vi "Calib_Substring_code.vi"(0 "Inst type":T1=enum."Pressure Transducer") -> (1 "Substring Type":string, 2 "Read file":bool)   [LabVIEW 2010]
uses:
  Controls/Inst_type.ctl
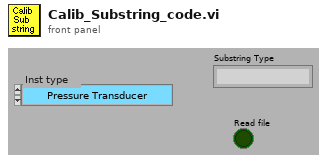
[diagram p1: front panel]
types:
  T1 = typedef "Inst_type.ctl" = enum16{"Propeller anemometer", "Raw voltage", "Pressure Transducer", "Pitot-static tube", "Preston tube", "Hot wire", "Cross wire 1", "Cross wire 2", "Generic Linear", "Generic Polynomial", "Generic BackPoly", "Fast FID", "Thermocouple", "Cold wire", "Pulsed Wire", "LDA Vel", "LDA Tran time", "LDA Arr time"}
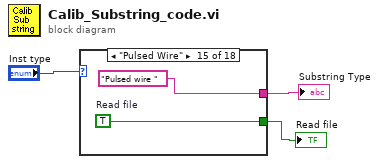
[diagram p0: block diagram]
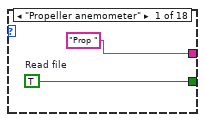
[diagram p2: hidden frame]
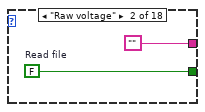
[diagram p3: hidden frame]
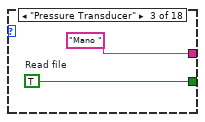
[diagram p4: hidden frame]
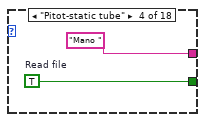
[diagram p5: hidden frame]
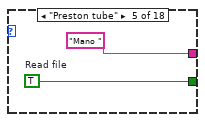
[diagram p6: hidden frame]
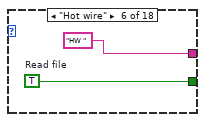
[diagram p7: hidden frame]
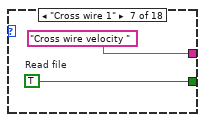
[diagram p8: hidden frame]
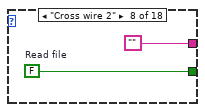
[diagram p9: hidden frame]
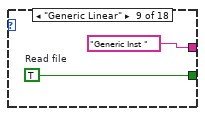
[diagram p10: hidden frame]
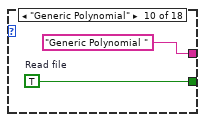
[diagram p11: hidden frame]
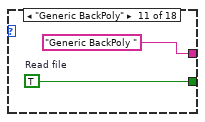
[diagram p12: hidden frame]
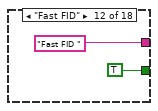
[diagram p13: hidden frame]
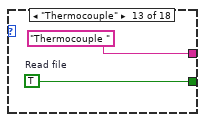
[diagram p14: hidden frame]
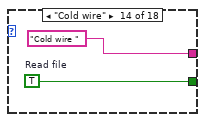
[diagram p15: hidden frame]
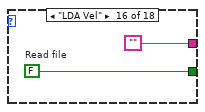
[diagram p16: hidden frame]
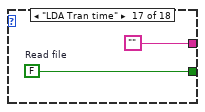
[diagram p17: hidden frame]
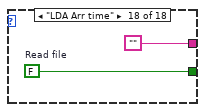
[diagram p18: hidden frame]
diagram:
  n1 = case shown="\"Pulsed Wire\"" "Inst type" {
    tunnel: [w5 w7 w9 w11 w13 w15 w17 w19 w21 w23 w25 TRUE ("Read file") w29 w31 w33 w35 w37 w39] -> w1
    tunnel: ["Prop " "" "Mano " "Mano " "Mano " "HW " "Cross wire velocity " "" "Generic Inst " "Generic Polynomial " "Generic BackPoly " "Fast FID " "Thermocouple " "Cold wire " "Pulsed wire " "" "" ""] -> w2
    frame "Propeller anemometer" {
      w5 = TRUE  # Read file
    }
    frame "Raw voltage" {
      w7 = FALSE  # Read file
    }
    frame "Pressure Transducer" {
      w9 = TRUE  # Read file
    }
    frame "Pitot-static tube" {
      w11 = TRUE  # Read file
    }
    frame "Preston tube" {
      w13 = TRUE  # Read file
    }
    frame "Hot wire" {
      w15 = TRUE  # Read file
    }
    frame "Cross wire 1" {
      w17 = TRUE  # Read file
    }
    frame "Cross wire 2" {
      w19 = FALSE  # Read file
    }
    frame "Generic Linear" {
      w21 = TRUE  # Read file
    }
    frame "Generic Polynomial" {
      w23 = TRUE  # Read file
    }
    frame "Generic BackPoly" {
      w25 = TRUE  # Read file
    }
    frame "Fast FID" {
    }
    frame "Thermocouple" {
      w29 = TRUE  # Read file
    }
    frame "Cold wire" {
      w31 = TRUE  # Read file
    }
    frame "Pulsed Wire" {
      w33 = TRUE  # Read file
    }
    frame "LDA Vel" {
      w35 = FALSE  # Read file
    }
    frame "LDA Tran time" {
      w37 = FALSE  # Read file
    }
    frame "LDA Arr time" {
      w39 = FALSE  # Read file
    }
  }
  "Substring Type" <- w2
  "Read file" <- w1
